vi "7p1_HW_Task1A_doanbs.vi"(10 "th, Theta in":dbl, 11 "Units in":string) -> (2 "th, Theta out":dbl, 3 "Units out":string)   [LabVIEW 2016]
uses:
  <vilib>/express/express arith-compare/Formula/XNode/ExpressFormulaBlockNode.xnode
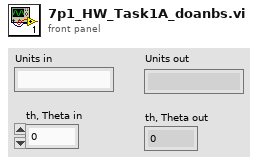
[diagram p1: front panel]
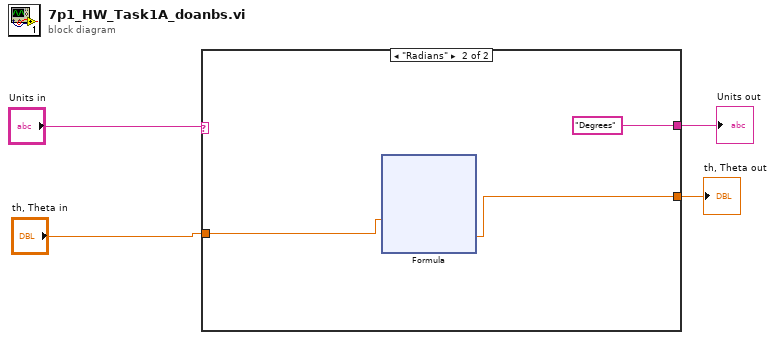
[diagram p0: block diagram]
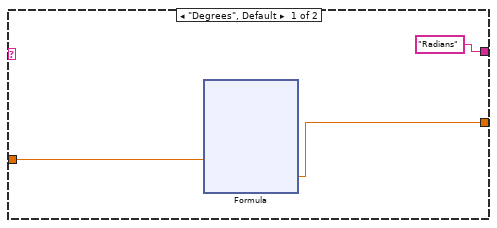
[diagram p2: hidden frame]
diagram:
  n1 = case shown="\"Radians\"" "Units in" {
    tunnel: "th, Theta in" -> [w7 w18]
    tunnel: ["Radians" "Degrees"] -> w3
    tunnel: [w5 w17] -> w4
    frame "Degrees", Default {
      n2 = xnode "Formula"("th"=w7) -> ("Result"=w5:dbl)  [unwired: 1 in, 1 out]
    }
    frame "Radians" {
      n3 = xnode "Formula"("th"=w18) -> ("Result"=w17:dbl)  [unwired: 1 in, 1 out]
    }
  }
  "Units out" <- w3
  "th, Theta out" <- w4
